vi "NotifyIcon Class Example.vi"() -> ()   [LabVIEW 2016]
doc: "This VI shows how to use the NotifyIcon Class VIs to create a simple Notification Icon and the associated Context Menu. Refer to the subdiagram and descriptions of the subVIs for an explanation of each function in the example.\n\n\nStinus Olsen\nCIM Industrial Systems A/S\n22. Feb. 2011 15:05\nmailto: seo@cim.as"
uses:
  Public/Controls/Notify Event Type.ctl
  Public/Tray Icon/Set Tray Notification Icon Poly/Set Tray Icon (string).vi
  Public/Tray Icon/Set Tray Notification Icon Poly/Set Tray Icon (file).vi
  NotifyIcon.lvclass
panel:
  in  "Set Tray Icon Tip Strip Text":string="This is the standard Tray Icon Tip text.."
  in  "boolPropBarBreak":bool caption="BarBreak"
  in  "boolPropChecked":bool caption="Checked"
  in  "boolPropVisible":bool=TRUE caption="Visible"
  in  "boolPropEnabled":bool=TRUE caption="Enabled"
  in  "boolPropDefaultItem":bool caption="Default Item"
  in  "strPropNodeTag":string="MNU_Inserted" caption="Item Tag"
  in  "btnSetProperty":bool
  in  "BalloonTip Icon":i32(ring)=1 items=["None", "Info", "Warning", "Error"]
  in  "Timeout (ms)":i32=5000
  in  "strTooltipTitle":string="Notify Icon Test Shell" caption="BalloonTip Title"
  in  "strTooltipText":string="This is the standard Balloon Tip Text.." caption="BalloonTip Text"
  in  "btnShowTooltip":bool
  in  "btnDeleteMenu":bool
  in  "strDelNodeTag":string="MNU_Inserted" caption="Item Tag"
  in  "iAddIndex":i32=-1 caption="Index"
  in  "strAddNodeText":string="New Menu Item" caption="Item Text"
  in  "Item Tag":string="MNU_Inserted"
  in  "strAddParentNodeTag":string caption="Parent Item Tag (root)"
  in  "btnAddMenu":bool
  in  "Icon File":path caption="(The input image is automatically resized to fit)"
  out "Notify Icon Event":T1
  in  "Set Tray Icon Visibility":bool=TRUE
  out "error out":errorcluster
  in  "btnExit":bool
  # "Notify Icon"
  # "Control the Tray Icon"
  # "Control the Tray Icon BalloonTip"
  # "Control the Context Menu"
  # "Delete Context Menu Item"
  # "Insert Context Menu Item"
  # "Change the Tray Icon"
  # "Context Menu Item Properties"
  # "Fig.3 A Context Menu example"
  # "Fig.2 Tray Icon BalloonTip example"
  # "To change the icon associated with the context menu in the notification area, select any BMP, GIF, JPG, PNG, TIFF or ICO file in the Path control below:"
  # "Fig.1 Notification Area Icons"
  # "Context Menu Items are based on Tags (unique strings) like the native LabVIEW Runtime Menu. Items can be linked to each other in a hierachy by using the Parent Tag property.\nIf the Parent Tag is left empty, the item will be added to the root of the menu.\n\nAdding an item with the text \"-\" will insert a separator line (a unique tag is still needed). A special VI is provided to insert separator lines.\n\nUse the ampersand (&) character in the item text to define the next character as the mnemonic for that Menu Item.\n\nInsert index:\nWhen inserting a new item, the insert index can be entered as well.\nIf the index is negative, the item will always be inserted as the last one (default), otherwise the index will be honored with respect to the current menu."
  # "Minimize & Close to Tray:\n\nPressing the Minimize or Close Window\nbuttons causes the VI to hide the FP.\nDoubleClick the Tray Icon to restore the\nVI Front Panel window.\n\nIf the Tray Icon is hidden when closing\nor minimizing the FP window, it will be\nunhidden to allow you to click it!"
  # "Generated Context Menu Event"
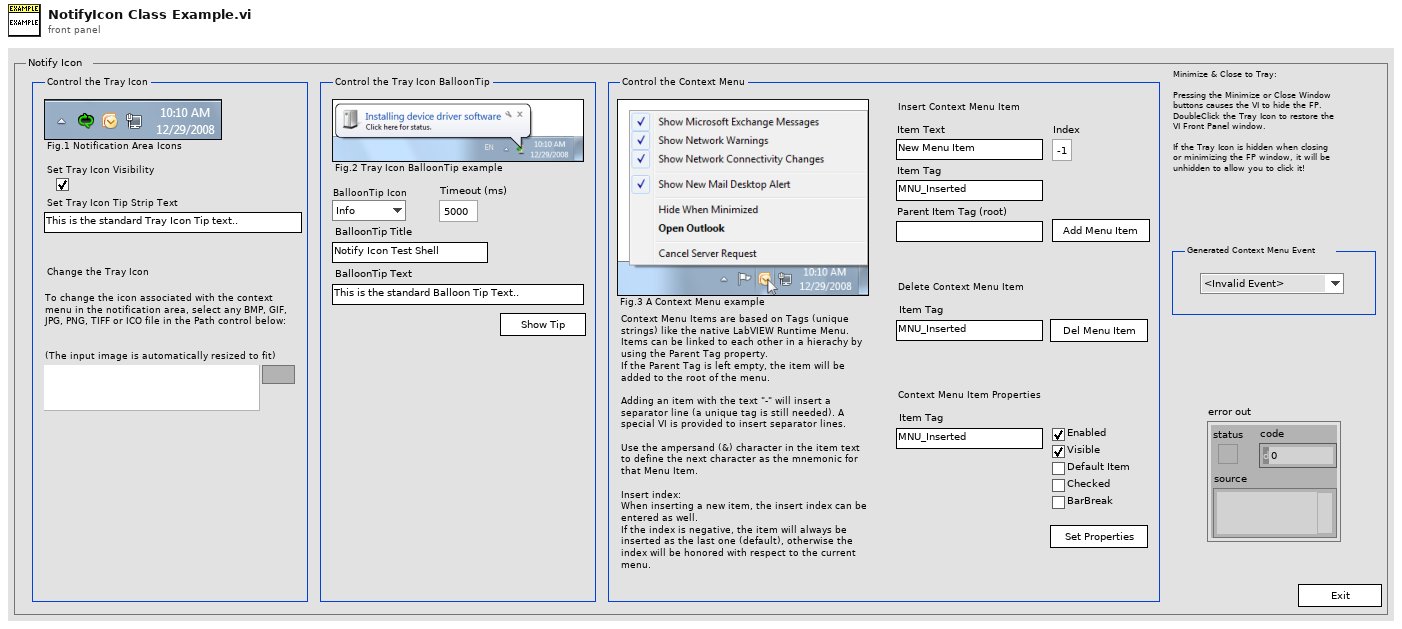
[diagram p1: front panel]
types:
  T1 = typedef "NotifyIcon.lvclass/Notify Event Type.ctl" = enum16{"<Invalid Event>", "Tray Icon Click", "Tray Icon DoubleClick", "BalloonTip Shown", "BalloonTip Clicked", "BalloonTip Closed", "Menu Item Clicked"}
  T2 = enum32{"Invalid", "Standard", "Closed", "Hidden", "Minimized", "Maximized"}
  T3 = typedef "sizeaction.ctl" = enum32{"Minimized", "Maximized", "Resized"}
  T4 = typedef "Notify Icon.lvclass/Notify Event Type.ctl" = enum16{"<Invalid Event>", "Tray Icon Click", "Tray Icon DoubleClick", "BalloonTip Shown", "BalloonTip Clicked", "BalloonTip Closed", "Menu Item Clicked"}
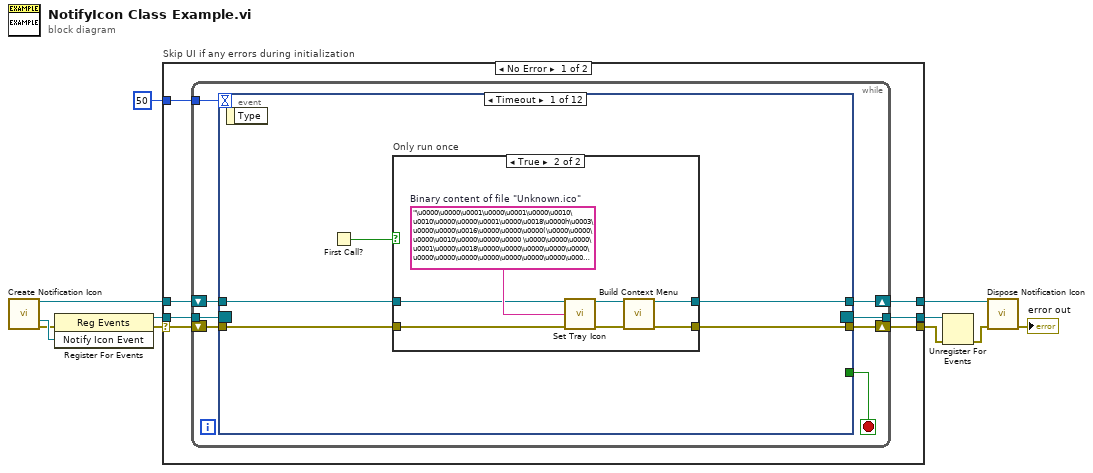
[diagram p0: block diagram]
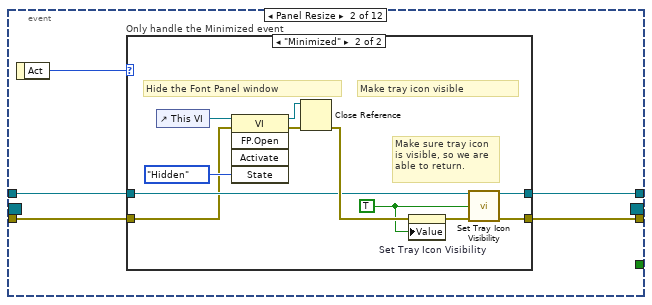
[diagram p3: hidden frame]
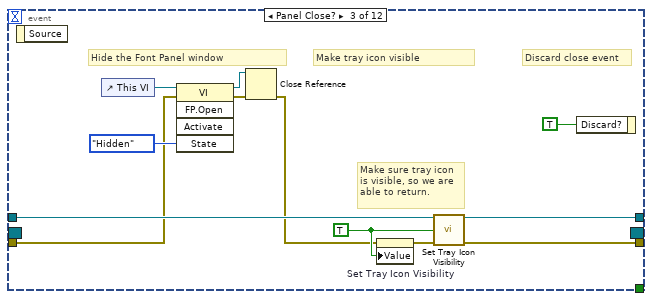
[diagram p5: hidden frame]
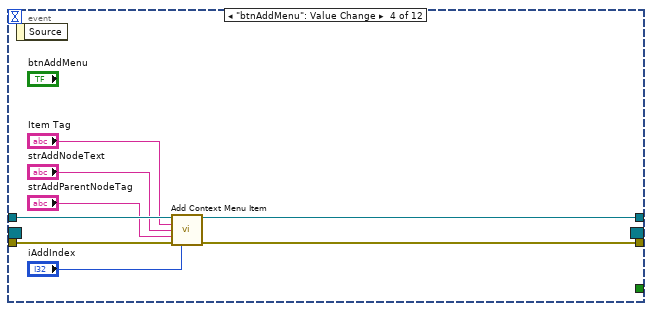
[diagram p6: hidden frame]
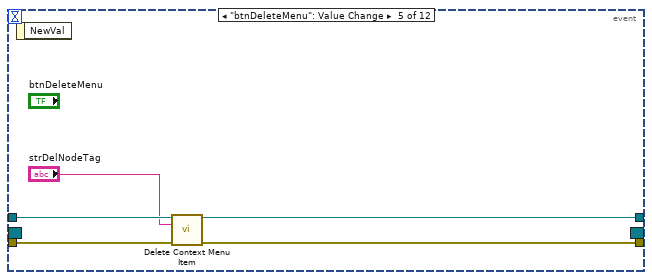
[diagram p7: hidden frame]
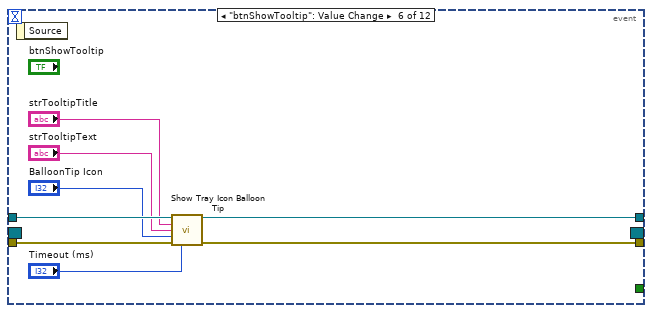
[diagram p8: hidden frame]
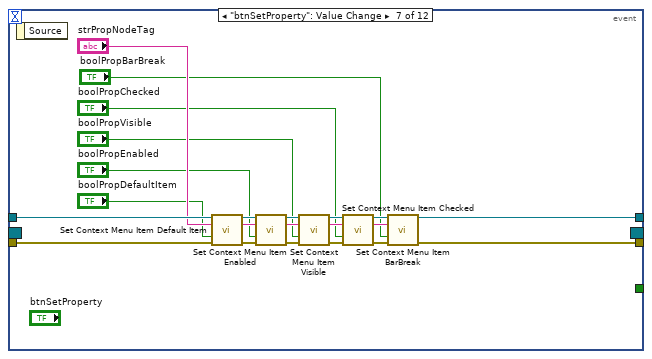
[diagram p9: hidden frame]
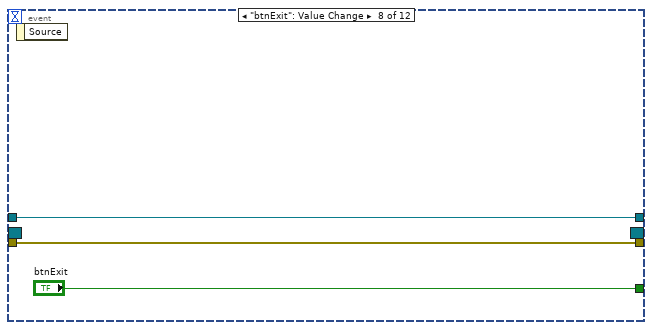
[diagram p10: hidden frame]
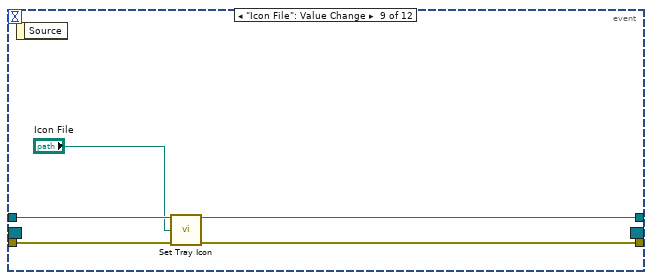
[diagram p11: hidden frame]
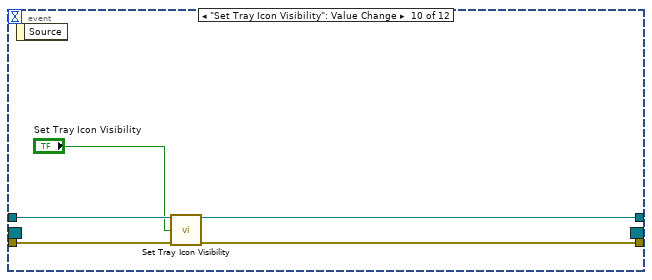
[diagram p12: hidden frame]
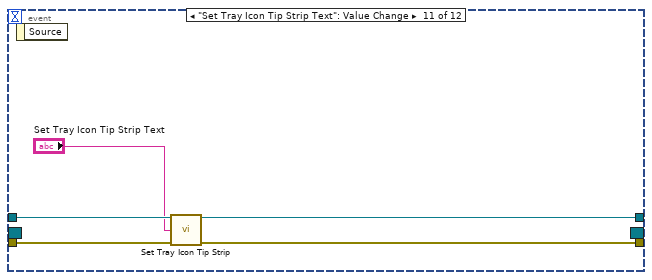
[diagram p13: hidden frame]
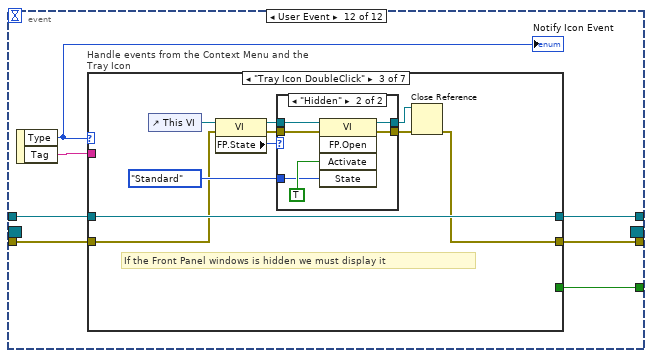
[diagram p14: hidden frame]
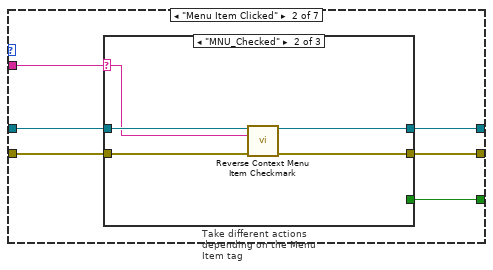
[diagram p16: hidden frame]
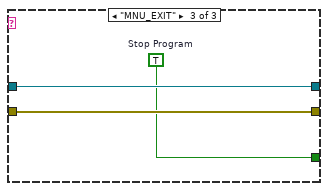
[diagram p18: hidden frame]
diagram:
  n1 = call "Create Notification Icon.vi"() -> ("NotifyIcon out"=w3:refnum<class "NotifyIcon.lvclass">, "Notify Icon Event"=w11:refnum<user-event>, "error out"=w2:errorcluster)  [unwired: 1 in, 12 out]
  n2 = register-events(error in=w2, w11) -> (reference out=w10:refnum<event-registration>, error out=w4:errorcluster)  [unwired: 1 in]
  n3 = case "Skip UI if any errors during initialization" shown="No Error" w4 {
    selector: w4 -> [w13 w183]
    tunnel: w10 -> [w18 w184]
    tunnel: [w17 w184] -> w9
    tunnel: [w16 w183] -> w8
    tunnel: w3 -> [w15 w185]
    tunnel: [w14 w185] -> w7
    tunnel: 50 -> [w12 _]
    frame No Error {
      n4 = while {
        shift-right: [w23] -> w16
        shift-left: w13 -> [w25]
        tunnel: w18 -> [w26]
        tunnel: [w24] -> w17
        shift-right: [w21] -> w14
        shift-left: w15 -> [w22]
        tunnel: w12 -> [w19]
        stop <- w20 stop-if-true
        n5 = event shown="[0] Timeout" {
          selector: w26 -> [_ _ _ _ _ _ _ _ _ _ _ _]
          dyn-events: [_ _ _ _ _ _ _ _ _ _ _ _] -> w24
          timeout: w19 -> [_ _ _ _ _ _ _ _ _ _ _ _]
          tunnel: w25 -> [w29 w41 w59 w78 w83 w90 w111 w116 w120 w124 w131 w135]
          tunnel: [w27 w42 w67 w71 w79 w89 w92 w116 w117 w123 w129 w133] -> w23
          tunnel: w22 -> [w31 w44 w65 w77 w82 w91 w113 w115 w121 w126 w128 w136]
          tunnel: [w28 w43 w66 w72 w80 w88 w93 w115 w118 w125 w130 w134] -> w21
          tunnel: [_ _ _ _ _ _ _ "btnExit" _ _ _ w132] -> w20
          event Timeout {
            n6 = event-data() -> ()  [unwired: 2 out]
            n7 = First Call?() -> (First Call?: T/F=w30:bool)
            n8 = case "Only run once" shown="True" w30 {
              tunnel: w31 -> [w33 w37]
              tunnel: w29 -> [w32 w36]
              tunnel: [w33 w35] -> w28
              tunnel: [w32 w34] -> w27
              frame False {
              }
              frame True {
                w40 = "\u0000\u0000\u0001\u0000\u0001\u0000\u0010\u0010\u0000\u0000\u0001\u0000\u0018\u0000h\u0003\u0000\u0000\u0016\u0000\u0000\u0000(\u0000\u0000\u0000\u0010\u0000\u0000\u0000 \u0000\u0000\u0000\u0001\u0000\u0018\u0000\u0000\u0000\u0000\u0000\u0000\u0000\u0000\u0000\u0000\u0000\u0000\u0000\u0000\u0000\u0000\u0000\u0000\u0000\u0000\u0000\u0000\u0000\u0000\u0000ÿÿÿÿÿÿÿÿÿÿÿÿÿÿÿÿÿÿÿÿÿÿÿÿÿÿÿÿÿÿÿÿÿÿÿÿÿÿÿÿÿÿÿÿÿÿÿÿÿÿÿww}PPvFFvDDrBBp@@n==l;;k::k::k99j99k<<vvÿÿÿÿÿÿVV£xx]]__]]XX__WWOONN}JJxEEn;;j;;ÿÿÿÿÿÿ__­iikkgg½ùôôûîî¯}}YYWWQQxEEi88ÿÿÿÿÿÿcc´£pp£pphhË¾¾ùÿÿÿÿÿÖ³³^^\\\\WW}JJi88ÿÿÿÿÿÿhh»©uu©vv©vvcc·À¢llhhbb^^NNj99ÿÿÿÿÿÿkkÄ¯zz°}}¯{{¾Á¹¤oollggbbTTk::ÿÿÿÿÿÿppÉ¢¢¶¶´Ñ°°ÿÿÿÿÿÿÇ¡llkkhhWWn==ÿÿÿÿÿÿttÑ««¼¾¼¹øõõÿÿÿÿÿÿÜºº¢llii\\\\rAAÿÿÿÿÿÿ¡xxÖ±±ÃÄÅ²zz³zzõîîÿÿÿÿÿÿ·ll__sBBÿÿÿÿÿÿ¤||Ü¹¹ÉÇ«}}ÞÙÙÐ¸¸ðììúûûÿÿÿ» mm``vFFÿÿÿÿÿÿ§~~à¿¿Ì..."  # Binary content of file "Unknown.ico"
                n9 = call-poly "Set Tray Icon.vi"("NotifyIcon in"=w37, "Icon String"=w40, "error in (no error)"=w36) -> ("NotifyIcon out"=w38:refnum<class "NotifyIcon.lvclass">, "error out"=w39:errorcluster)  [unwired: 11 out]
                n10 = call "Build Context Menu.vi"("NotifyIcon in"=w38, "error in (no error)"=w39) -> ("NotifyIcon out"=w35:refnum<class "NotifyIcon.lvclass">, "error out"=w34:errorcluster)  [unwired: 12 out]
              }
            }
          }
          event Panel Resize {
            n11 = event-data() -> ("Act"=w45:T3)  [unwired: 1 out]
            n12 = case "Only handle the Minimized event" shown="\"Minimized\"" w45 {
              tunnel: w44 -> [w47 w53]
              tunnel: [w47 w52] -> w43
              tunnel: [w46 w49] -> w42
              tunnel: w41 -> [w46 w48]
              frame Default {
              }
              frame "Minimized" {
                w50 = TRUE
                # "Make tray icon visible"
                # "Hide the Font Panel window"
                # "Make sure tray icon\nis visible, so we are\nable to return."
                n13 = control-ref of="This VI"() -> (w55:refnum<vi>)
                n14 = invoke class="VI" method="FP.Open"(reference=w55, error in=w48, "State"=T2."Hidden") -> (reference out=w56:refnum<vi>, error out=w57:errorcluster)  [unwired: 2 in, 3 out]
                n15 = Close Reference(reference=w56, error in (no error)=w57) -> (error out=w54:errorcluster)
                n16 = property on="Set Tray Icon Visibility" class="Bool (strict)"(error in=w54, "Value"=w50) -> (error out=w51:errorcluster)  [unwired: 1 in, 1 out]
                n17 = call "Set Tray Icon Visibility.vi"("NotifyIcon in"=w53, "Show Tray Icon"=w50, "error in (no error)"=w51) -> ("NotifyIcon out"=w52:refnum<class "NotifyIcon.lvclass">, "error out"=w49:errorcluster)  [unwired: 11 out]
              }
            }
          }
          event Panel Close? {
            w68 = TRUE
            # "Hide the Font Panel window"
            # "Discard close event"
            # "Make tray icon visible"
            # "Make sure tray icon\nis visible, so we are\nable to return."
            n18 = event-data() -> ()  [unwired: 2 out]
            n19 = control-ref of="This VI"() -> (w64:refnum<vi>)
            n20 = invoke class="VI" method="FP.Open"(reference=w64, error in=w59, "State"=T2."Hidden") -> (reference out=w63:refnum<vi>, error out=w62:errorcluster)  [unwired: 2 in, 3 out]
            n21 = Close Reference(reference=w63, error in (no error)=w62) -> (error out=w60:errorcluster)
            n22 = property on="Set Tray Icon Visibility" class="Bool (strict)"(error in=w60, "Value"=w68) -> (error out=w69:errorcluster)  [unwired: 1 in, 1 out]
            n23 = call "Set Tray Icon Visibility.vi"("NotifyIcon in"=w65, "Show Tray Icon"=w68, "error in (no error)"=w69) -> ("NotifyIcon out"=w66:refnum<class "NotifyIcon.lvclass">, "error out"=w67:errorcluster)  [unwired: 11 out]
            n24 = event-data("Discard?"=TRUE) -> ()  [unwired: 1 in, 1 out]
          }
          event "btnAddMenu": Value Change {
            n25 = event-data() -> ()  [unwired: 2 out]
            n26 = call "Add Context Menu Item.vi"("NotifyIcon in"=w77, "Item Tag"="Item Tag", "Item Text"="strAddNodeText", "Parent Item Tag (\"\")"="strAddParentNodeTag", "error in (no error)"=w78, "Item Index (Last)"="iAddIndex") -> ("NotifyIcon out"=w72:refnum<class "NotifyIcon.lvclass">, "error out"=w71:errorcluster)  [unwired: 8 out]
          }
          event "btnDeleteMenu": Value Change {
            n27 = event-data() -> ()  [unwired: 2 out]
            n28 = call "Delete Context Menu Item.vi"("NotifyIcon in"=w82, "Item Tag"="strDelNodeTag", "error in (no error)"=w83) -> ("NotifyIcon out"=w80:refnum<class "NotifyIcon.lvclass">, "error out"=w79:errorcluster)  [unwired: 11 out]
          }
          event "btnShowTooltip": Value Change {
            n29 = event-data() -> ()  [unwired: 2 out]
            n30 = call "Show Tray Icon Balloon Tip.vi"("NotifyIcon in"=w91, "Title"="strTooltipTitle", "Text"="strTooltipText", "Icon"="BalloonTip Icon", "error in (no error)"=w90, "Timeout (ms)"="Timeout (ms)") -> ("NotifyIcon out"=w88:refnum<class "NotifyIcon.lvclass">, "error out"=w89:errorcluster)  [unwired: 8 out]
          }
          event "btnSetProperty": Value Change {
            n31 = event-data() -> ()  [unwired: 2 out]
            n32 = call "Set Context Menu Item Default Item.vi"("NotifyIcon in"=w113, "Item Tag"="strPropNodeTag", "Default Item (False)"="boolPropDefaultItem", "error in (no error)"=w111) -> ("NotifyIcon out"=w109:refnum<class "NotifyIcon.lvclass">, "dub Item Tag"=w107:string, "error out"=w108:errorcluster)  [unwired: 9 out]
            n33 = call "Set Context Menu Item Enabled.vi"("NotifyIcon in"=w109, "Item Tag"=w107, "Enabled (True)"="boolPropEnabled", "error in (no error)"=w108) -> ("NotifyIcon out"=w105:refnum<class "NotifyIcon.lvclass">, "dub Item Tag"=w103:string, "error out"=w104:errorcluster)  [unwired: 9 out]
            n34 = call "Set Context Menu Item Visible.vi"("NotifyIcon in"=w105, "Item Tag"=w103, "Visible (True)"="boolPropVisible", "error in (no error)"=w104) -> ("NotifyIcon out"=w101:refnum<class "NotifyIcon.lvclass">, "dub Item Tag"=w99:string, "error out"=w100:errorcluster)  [unwired: 9 out]
            n35 = call "Set Context Menu Item Checked.vi"("NotifyIcon in"=w101, "Item Tag"=w99, "Checked (False)"="boolPropChecked", "error in (no error)"=w100) -> ("NotifyIcon out"=w96:refnum<class "NotifyIcon.lvclass">, "dub Item Tag"=w95:string, "error out"=w97:errorcluster)  [unwired: 9 out]
            n36 = call "Set Context Menu Item BarBreak.vi"("NotifyIcon in"=w96, "Item Tag"=w95, "BarBreak (False)"="boolPropBarBreak", "error in (no error)"=w97) -> ("NotifyIcon out"=w93:refnum<class "NotifyIcon.lvclass">, "error out"=w92:errorcluster)  [unwired: 10 out]
          }
          event "btnExit": Value Change {
            n37 = event-data() -> ()  [unwired: 2 out]
          }
          event "Icon File": Value Change {
            n38 = event-data() -> ()  [unwired: 2 out]
            n39 = call-poly "Set Tray Icon.vi"("NotifyIcon in"=w121, "Image file"="Icon File", "error in (no error)"=w120) -> ("NotifyIcon out"=w118:refnum<class "NotifyIcon.lvclass">, "error out"=w117:errorcluster)  [unwired: 11 out]
          }
          event "Set Tray Icon Visibility": Value Change {
            n40 = event-data() -> ()  [unwired: 2 out]
            n41 = call "Set Tray Icon Visibility.vi"("NotifyIcon in"=w126, "Show Tray Icon"="Set Tray Icon Visibility", "error in (no error)"=w124) -> ("NotifyIcon out"=w125:refnum<class "NotifyIcon.lvclass">, "error out"=w123:errorcluster)  [unwired: 11 out]
          }
          event "Set Tray Icon Tip Strip Text": Value Change {
            n42 = event-data() -> ()  [unwired: 2 out]
            n43 = call "Set Tray Icon Tip Strip.vi"("NotifyIcon in"=w128, "Icon Tip Strip Text"="Set Tray Icon Tip Strip Text", "error in (no error)"=w131) -> ("NotifyIcon out"=w130:refnum<class "NotifyIcon.lvclass">, "error out"=w129:errorcluster)  [unwired: 11 out]
          }
          event User Event {
            n44 = event-data() -> ("Type"=w138:T4, "Tag"=w137:string)  [unwired: 1 out]
            "Notify Icon Event" <- w138
            n45 = case "Handle events from the Context Menu and the Tray Icon" shown="\"Tray Icon DoubleClick\"" w138 {
              tunnel: w137 -> [_ w145 _ _ _ _ _]
              tunnel: w136 -> [w140 w146 w166 w176 w178 w180 w182]
              tunnel: w135 -> [w139 w144 w158 w175 w177 w179 w181]
              tunnel: [w140 w143 w166 w176 w178 w180 w182] -> w134
              tunnel: [w139 w142 w157 w175 w177 w179 w181] -> w133
              tunnel: [_ w141 _ _ _ _ _] -> w132
              frame "<Invalid Event>", Default {
              }
              frame "Menu Item Clicked" {
                n46 = case "Take different actions depending on the Menu Item tag" shown="\"MNU_Checked\"" w145 {
                  selector: w145 -> [_ w149 _]
                  tunnel: w146 -> [w148 w151 w156]
                  tunnel: w144 -> [w147 w153 w155]
                  tunnel: [w148 w150 w156] -> w143
                  tunnel: [w147 w152 w155] -> w142
                  tunnel: [_ _ w154] -> w141
                  frame "False", Default {
                  }
                  frame "MNU_Checked" {
                    n47 = call "Reverse Context Menu Item Checkmark.vi"("NotifyIcon in"=w151, "Item Tag"=w149, "error in (no error)"=w153) -> ("NotifyIcon out"=w150:refnum<class "NotifyIcon.lvclass">, "error out"=w152:errorcluster)  [unwired: 11 out]
                  }
                  frame "MNU_EXIT" {
                    w154 = TRUE  # Stop Program
                  }
                }
              }
              frame "Tray Icon DoubleClick" {
                # "If the Front Panel windows is hidden we must display it"
                n48 = control-ref of="This VI"() -> (w165:refnum<vi>)
                n49 = property class="VI"(reference=w165, error in=w158) -> (reference out=w163:refnum<vi>, error out=w162:errorcluster, "FP.State"=w164:T2)
                n50 = case shown="\"Hidden\"" w164 {
                  tunnel: w163 -> [w168 w174]
                  tunnel: w162 -> [w167 w173]
                  tunnel: T2."Standard" ("State") -> [_ w171]
                  tunnel: [w167 w170] -> w160
                  tunnel: [w168 w169] -> w159
                  frame "Invalid", Default {
                  }
                  frame "Hidden" {
                    n51 = invoke class="VI" method="FP.Open"(reference=w174, error in=w173, "Activate"=TRUE, "State"=w171) -> (reference out=w169:refnum<vi>, error out=w170:errorcluster)  [unwired: 1 in, 3 out]
                  }
                }
                n52 = Close Reference(reference=w159, error in (no error)=w160) -> (error out=w157:errorcluster)
              }
              frame "BalloonTip Shown" {
              }
              frame "BalloonTip Clicked" {
              }
              frame "BalloonTip Closed" {
              }
              frame "Tray Icon Click" {
              }
            }
          }
        }
      }
    }
    frame Error {
    }
  }
  n53 = Unregister For Events(event registration refnum=w9, error in=w8) -> (error out=w6:errorcluster)
  n54 = call "Dispose Notification Icon.vi"("NotifyIcon in"=w7, "error in (no error)"=w6) -> ("error out"=→"error out":errorcluster)  [unwired: 13 out]
